vi "Get Oscillator Freq.vi"(10 "Reference Clock":dbl, 11 "Array 3":string[](array[string])) -> (0 "Reference Clock Multiplier":dbl[](array[numeric]), 1 "Oscillator Freqs":dbl[](array[numeric]), 2 "Scaling Factor":dbl[](array[numeric]), 3 "Tuning Word":string[](array[string]))   [LabVIEW 2018]
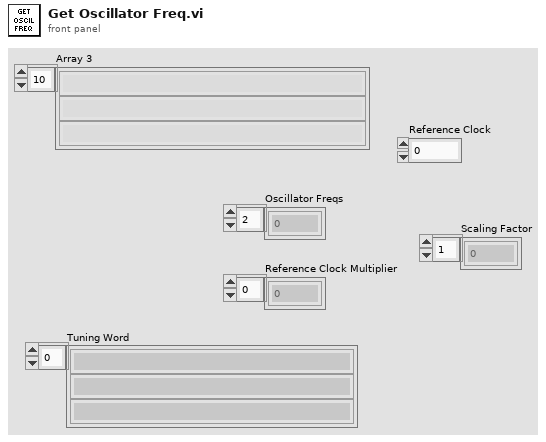
[diagram p1: front panel]
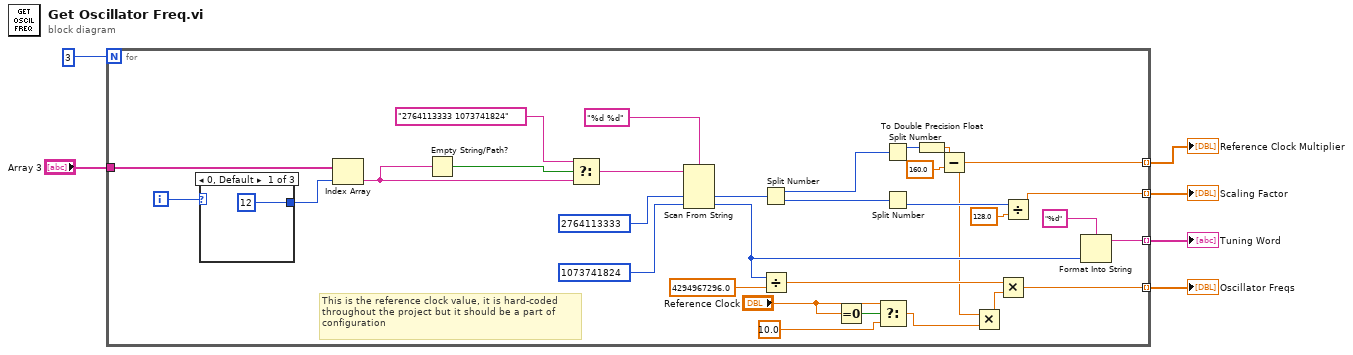
[diagram p0: block diagram]
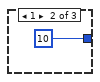
[diagram p2: hidden frame]
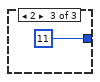
[diagram p3: hidden frame]
diagram:
  n1 = for {
    N: 3 -> [_]
    tunnel: "Array 3" -> [w36]
    tunnel: [w25] -> w6 mode=indexing
    tunnel: [w22] -> w5 mode=indexing
    tunnel: [w18] -> w2 mode=indexing
    tunnel: [w12] -> w1 mode=indexing
    i -> [w37]
    # "This is the reference clock value, it is hard-coded \nthroughout the project but it should be a part of\nconfiguration"
    n2 = case shown="0, Default" w37 {
      tunnel: [12 ("y") 10 ("y") 11 ("y")] -> w35
      frame 0, Default {
      }
      frame 1 {
      }
      frame 2 {
      }
    }
    n3 = Index Array(array=w36, index=w35) -> (element=w30:string)
    n4 = Empty String/Path?(string/path=w30) -> (empty?=w33:bool)
    n5 = Select(t="2764113333 1073741824", s=w33, f=w30) -> (s? t:f=w31:string)
    n6 = Scan From String(format string="%d %d", input string=w31, default 1=u32 2764113333 ("default value 1"), default 2=u32 1073741824 ("default value 1")) -> (output 1=w13:u32, output 2=w23:u32)  [unwired: 2 in, 3 out]
    n7 = Split Number(x=w13) -> (hi(x)=w17:u16, lo(x)=w21:u16)
    n8 = Divide(x=w23, y=4294967296.0) -> (x/y=w26:dbl)
    n9 = Equal To 0?(x="Reference Clock") -> (x = 0?=w8:bool)
    n10 = Select(t="Reference Clock", s=w8, f=10.0 ("y")) -> (s? t:f=w7:dbl)
    n11 = Split Number(x=w17) -> (hi(x)=w16:u8)  [unwired: 1 out]
    n12 = Split Number(x=w21) -> (lo(x)=w20:u8)  [unwired: 1 out]
    n13 = To Double Precision Float(number=w16) -> (double precision float=w15:dbl)
    n14 = Subtract(x=w15, y=160.0) -> (x-y=w12:dbl)
    n15 = Multiply(x=w12, y=w7) -> (x*y=w11:dbl)
    n16 = Multiply(x=w26, y=w11) -> (x*y=w25:dbl)
    n17 = Divide(x=w20, y=128.0) -> (x/y=w18:dbl)
    n18 = Format Into String(format string="%d", w23) -> (resulting string=w22:string)  [unwired: 2 in, 1 out]
  }
  "Oscillator Freqs" <- w6
  "Tuning Word" <- w5
  "Scaling Factor" <- w2
  "Reference Clock Multiplier" <- w1
